vi "LastErrorCluster.vi"() -> ()   [LabVIEW 2020]
panel:
  out "error out":errorcluster caption="Error Out"
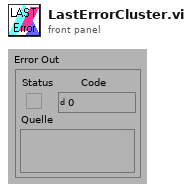
[diagram p1: front panel]
diagram:
